vi "Read Current Frame.vi"(8 "error in (no error)":errorcluster, 11 "Video Processor in":refnum<class "Video Cam Processor.lvclass">) -> (0 "error out":errorcluster, 2 "Video Frame.lvclass":refnum<class "Video Frame.lvclass">, 3 "Video Processor out":refnum<class "Video Cam Processor.lvclass">)   [LabVIEW 2018, in "Video Cam Processor.lvclass"]
uses:
  Video Cam Processor.lvclass
  Video Frame/Video Frame.lvclass
  Video Cam Processor.lvclass/Video Cam Processor.ctl
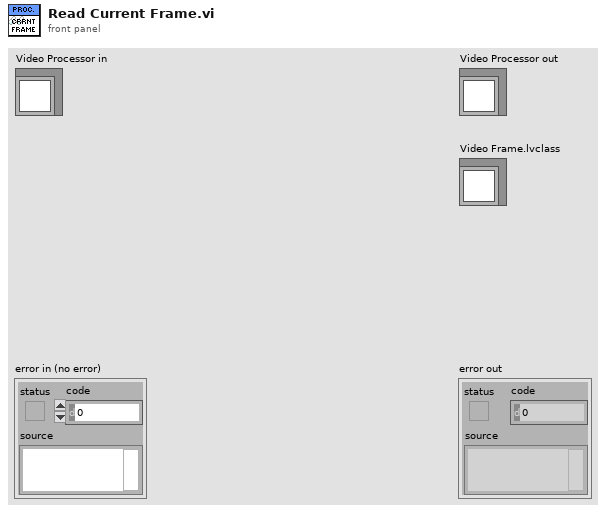
[diagram p1: front panel]
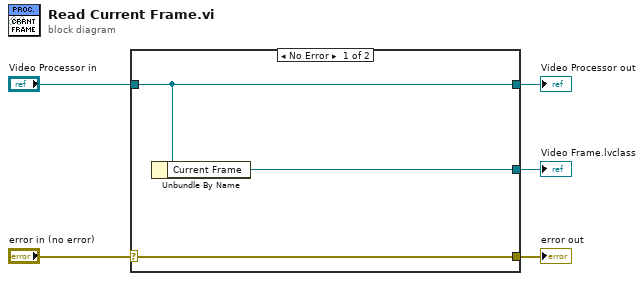
[diagram p0: block diagram]
diagram:
  n1 = case shown="No Error" "error in (no error)" {
    selector: "error in (no error)" -> [w8 w9]
    tunnel: [w8 w9] -> w4
    tunnel: [w7 w10] -> w2
    tunnel: "Video Processor in" -> [w7 w10]
    tunnel: [w6 _] -> w1
    frame No Error {
      n2 = Unbundle By Name(w7) -> ("Current Frame"=w6:refnum<class "Video Frame.lvclass">)
    }
    frame Error {
    }
  }
  "error out" <- w4
  "Video Processor out" <- w2
  "Video Frame.lvclass" <- w1
